vi "PKYK_Done_Checker.vi"(8 "error in (no error)":errorcluster, 11 "Ref in":T2={"MS SQL Connection"=refnum, "UDL File"=path "", "Time"="", "DCODE"="", "WIP+1"=0, "MC No?"=0, "POKAYOKE?"=FALSE, "Expected Result"="", "Result [Status]"="", "Clock"=0.0, "RFID"="", "WIP Queue"=refnum, "TS Parameter"={"ProfitCenterCode"="", "LineCode"="", "WorkOrderNumber"="", "Model"="", "Model_with_Prefix"="", "VendorCode"="", "SetParameterDateCode"="", "PokaYoke"=0, "Target"=1, "Live_DateCode"="", "CustomerPartNumber"="", "Hand"="", "sBarcode"=FALSE, "FCA"=0, "Ent_Stamp"=timestamp(0 s since 1904-01-01), "STS_CD"=0.0}, "Data_Queue"=[], "RFID Serial No."=""} {"TS Parameter"."FCA" format="%01d"; "TS Parameter"."Target" min=1 max=100000; "TS Parameter"."PokaYoke" min=0 max=1}) -> (0 "error out":errorcluster, 3 "Ref out":T2={"MS SQL Connection"=refnum, "UDL File"=path "", "Time"="", "DCODE"="", "WIP+1"=0, "MC No?"=0, "POKAYOKE?"=FALSE, "Expected Result"="", "Result [Status]"="", "Clock"=0.0, "RFID"="", "WIP Queue"=refnum, "TS Parameter"={"ProfitCenterCode"="", "LineCode"="", "WorkOrderNumber"="", "Model"="", "Model_with_Prefix"="", "VendorCode"="", "SetParameterDateCode"="", "PokaYoke"=0, "Target"=1, "Live_DateCode"="", "CustomerPartNumber"="", "Hand"="", "sBarcode"=FALSE, "FCA"=0, "Ent_Stamp"=timestamp(0 s since 1904-01-01), "STS_CD"=0.0}, "Data_Queue"=[], "RFID Serial No."=""} {"TS Parameter"."FCA" format="%01d"; "TS Parameter"."Target" min=1 max=100000; "TS Parameter"."PokaYoke" min=0 max=1}, 4 "Pokayoke Done?":bool, 5 "Expected Result":string, 7 "Pky Status":T1)   [LabVIEW 2020]
uses:
  Controls/TD SQL.ctl
  <vilib>/addons/database/Connection.llb/Conn ObjectReference.ctl
  Controls/WIP_State.ctl
  Controls/TS_Parameter.ctl
  Controls/Poka_Status.ctl
  MS SQL/MS_Global.vi
  <vilib>/addons/database/NI_Database_API.lvlib
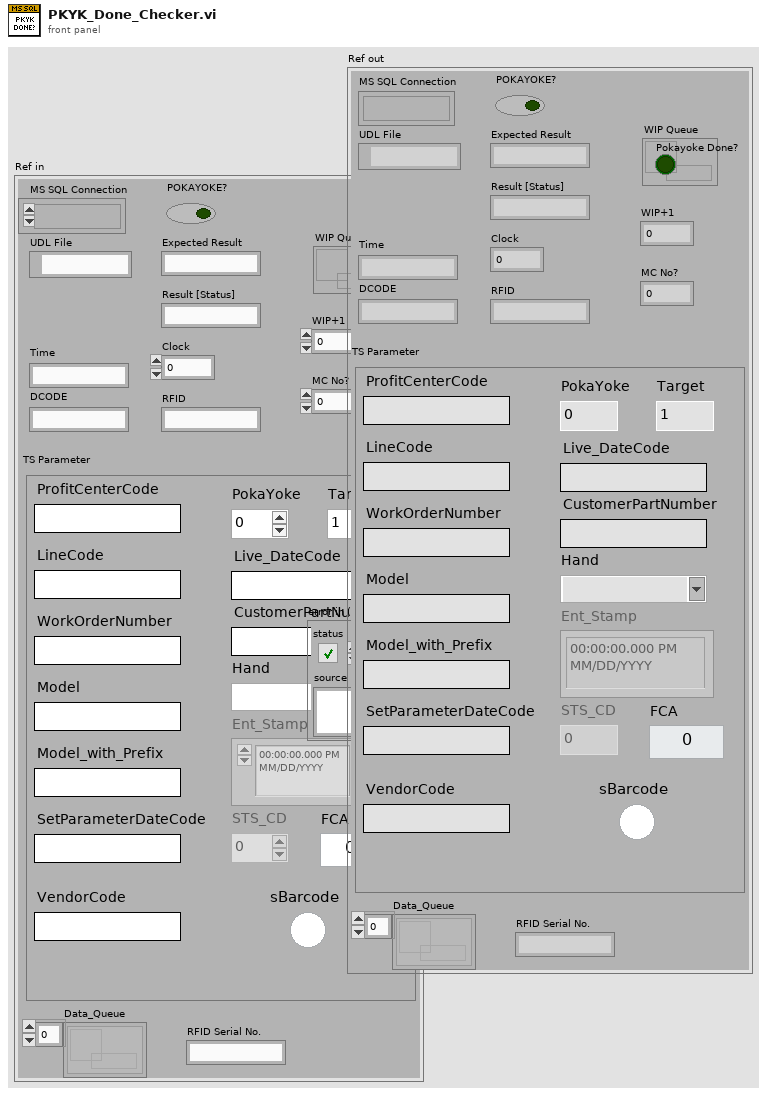
[diagram p1: front panel]
types:
  T1 = typedef "Poka_Status.ctl" = u16
  T2 = typedef "TD SQL.ctl" = cluster{"MS SQL Connection":T3, "UDL File":path, "Time":string, "DCODE":string, "WIP+1":i64, "MC No?":i32, "POKAYOKE?":bool, "Expected Result":string, "Result [Status]":string, "Clock":dbl, "RFID":string, "WIP Queue":refnum<queue>, "TS Parameter":T4, "Data_Queue":refnum<queue>[], "RFID Serial No.":string}
  T3 = typedef "NI_Database_API.lvlib/Conn ObjectReference.ctl" = refnum<k1>
  T4 = typedef "TS_Parameter.ctl" = cluster{"ProfitCenterCode":string, "LineCode":string, "WorkOrderNumber":string, "Model":string, "Model_with_Prefix":string, "VendorCode":string, "SetParameterDateCode":string, "PokaYoke":i32, "Target":i32, "Live_DateCode":string, "CustomerPartNumber":string, "Hand":string, "sBarcode":bool, "FCA":i32, "Ent_Stamp":timestamp, "STS_CD":dbl}
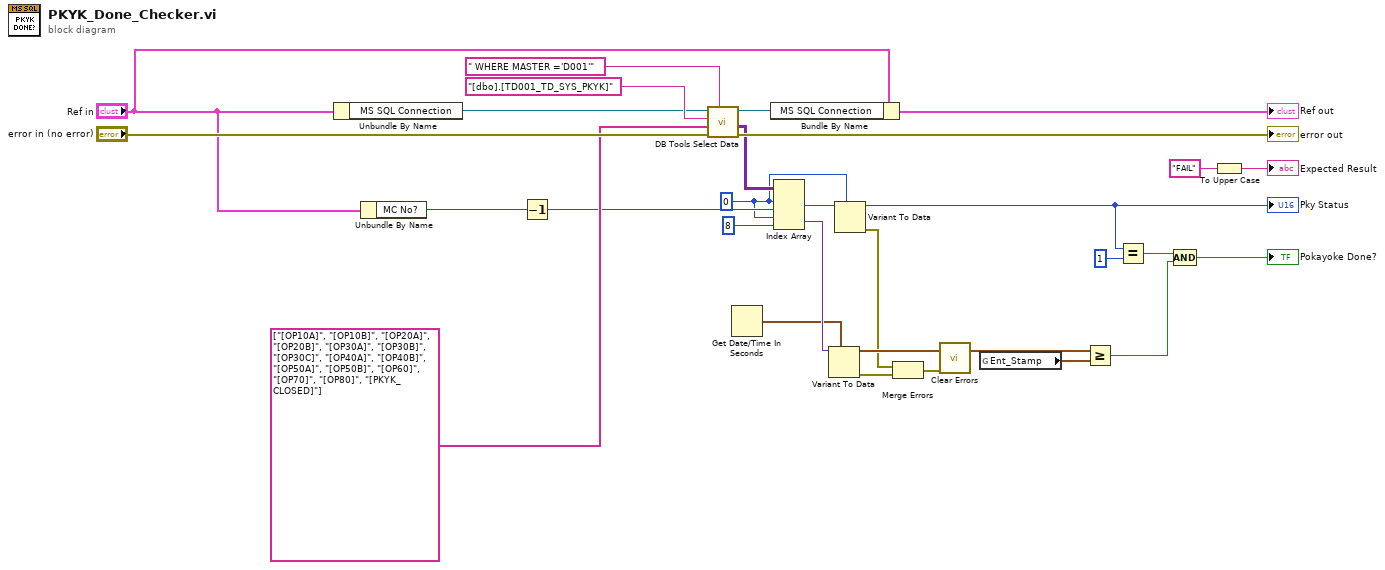
[diagram p0: block diagram]
diagram:
  w14 = 0 ("index (row)")
  n1 = Unbundle By Name("Ref in") -> ("MS SQL Connection"=w7:T3)
  n2 = Unbundle By Name("Ref in") -> ("MC No?"=w1:i32)
  n3 = Decrement(x=w1) -> (x-1=w15:i32)
  n4 = call <vilib>:"DB Tools Select Data.vi"("condition"=" WHERE MASTER ='D001'", "error in (no error)"="error in (no error)", "columns"=string[] ["[OP10A]", "[OP10B]", "[OP20A]", "[OP20B]", "[OP30A]", "[OP30B]", "[OP30C]", "[OP40A]", "[OP40B]", "[OP50A]", "[OP50B]", "[OP60]", "[OP70]", "[OP80]", "[PKYK_CLOSED]"] ("array 2"), "table"="[dbo].[TD001_TD_SYS_PKYK]", "connection reference"=w7) -> ("error out"=→"error out":errorcluster, "data"=w19:variant[][], "connection reference out"=w23:T3)  [unwired: 1 in]
  n5 = Get Date/Time In Seconds() -> (seconds since 1Jan1904=w11:timestamp)
  n6 = Bundle By Name(cluster="Ref in", "MS SQL Connection"=w23) -> (→"Ref out":T2)
  n7 = Index Array(array=w19, index (row) #1=w14, index (col) #1=w15, index (row) #2=w14, index (col) #2=8 ("disabled index (col)")) -> (element #1=w18:variant, element #2=w12:variant)
  n8 = Variant To Data(type=w11, Variant=w12) -> (data=w10:timestamp, error out=w5:errorcluster)  [unwired: 1 in]
  n9 = Variant To Data(type=w14, Variant=w18) -> (data=w24:i32, error out=w4:errorcluster)  [unwired: 1 in]
  "Pky Status" <- w24
  n10 = Merge Errors(w4, w5) -> (w3:errorcluster)
  n11 = call <vilib>:"Clear Errors.vi"("error in (no error)"=w3) -> ()  [unwired: 5 in, 2 out]
  n12 = global read "MS_Global.vi" "Ent_Stamp"() -> (w9:timestamp)
  n13 = Greater Or Equal?(x=w10, y=w9) -> (x >= y?=w8:bool)
  n14 = Equal?(x=w24, y=1) -> (x = y?=w16:bool)
  n15 = Compound Arithmetic op=AND(w16, w8) -> (→"Pokayoke Done?":bool)
  n16 = To Upper Case(1:"FAIL" ("string")) -> (0:→"Expected Result":string)
